vi "GEA2 Loop Check.vi"() -> ()   [LabVIEW 2016]
uses:
  LabVIEW GEA2 Toolkit v1.0.0.0/library/GEA2_Toolkit.lvlib
  HEWH/Type Definitions/GEA2 Commands.ctl
panel:
  out "min value":dbl
  out "max value":dbl
  out "Elapsed Time (sec)":dbl format="%.2f"
  in  "millisecond multiple":u32=1000
  out "T2(TankSensor)":dbl
  in  "stop":bool
  out "appended array":string[][](array[string])
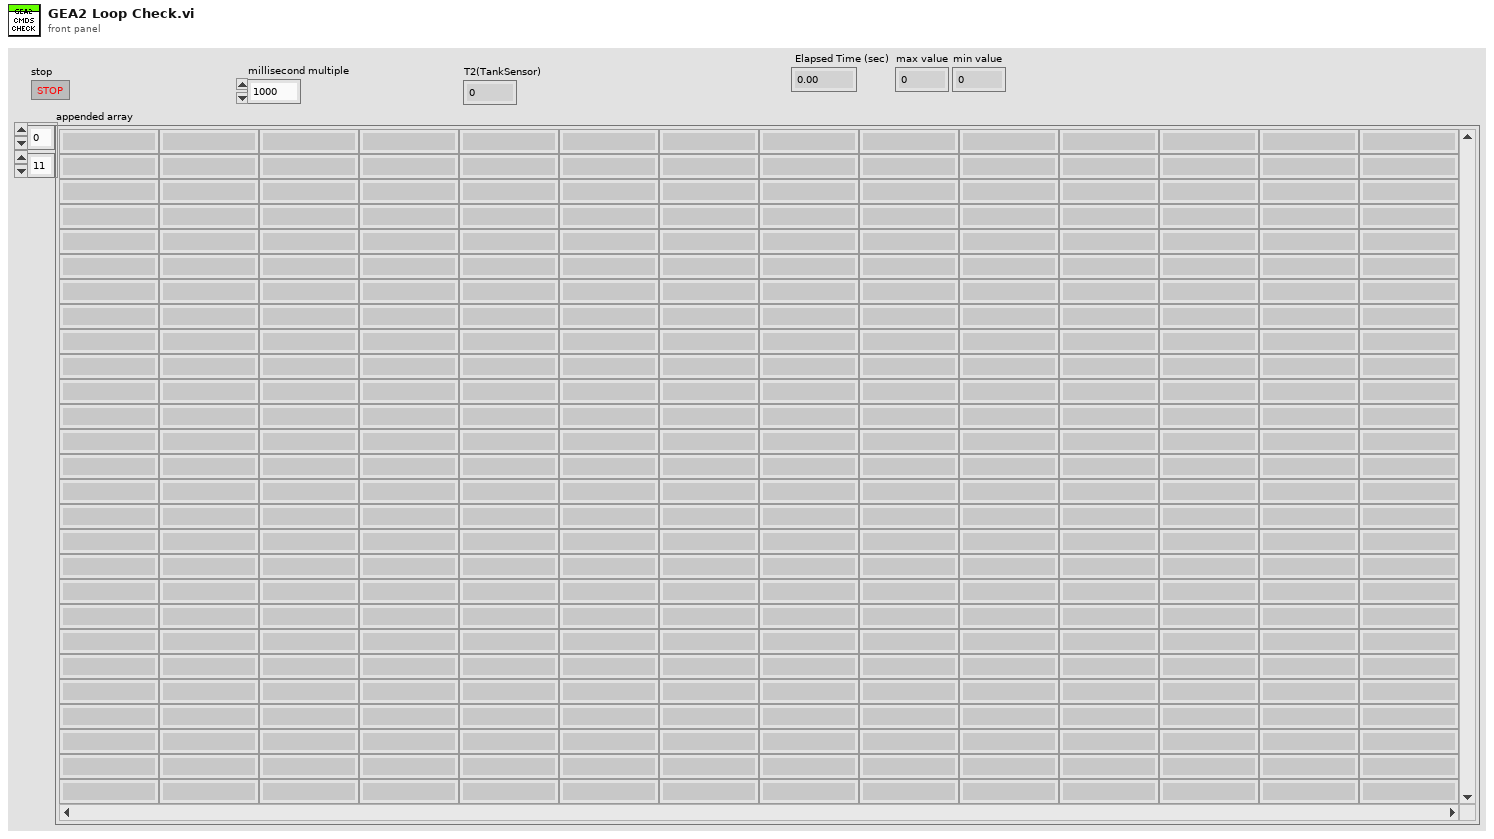
[diagram p1: front panel]
types:
  T1 = typedef "GEA2 Commands.ctl" = enum16{"CMD_CANCEL_EEV_POSITION", "CMD_CLEAR_ENERGY_USAGE_CTRS", "CMD_CLEAR_FAULT_COUNTS", "CMD_CLEAR_OVERRIDE_STATUS", "CMD_COMP_OFF", "CMD_COMP_ON", "CMD_DSM_OVERRIDES", "CMD_EEV_POSITION", "CMD_ENTER_EXIT_FCT_MODE", "CMD_ENTER_FACT_MODE", "CMD_HP_RUN_6MIN", "CMD_INITIATE_REMOTE_DSM_OVERRIDE", "CMD_LE_2_SECONDS", "CMD_REFRESH_SERVICE_TIMEOUTS", "CMD_RESET", "CMD_RESET_FILTER_TIMES", "CMD_RESTORE_EEPROM_DEFAULTS", "CMD_RQST_LED_STATUS", "CMD_SET_AMBIENT_THRESH_1", "CMD_SET_AMBIENT_THRESH_2", "CMD_SET_AMBIENT_THRESH_3", "CMD_SET_CURRENTS", "CMD_SET_EEV_DRIVE_LINES", "CMD_SET_EEV_STOP_POSITION", "CMD_SET_LEDS", "CMD_SET_MODEL_NUMBER", "CMD_SET_PID_I_DENOM_OVER_THR", "CMD_SET_PID_I_DENOM_UNDER_THR", "CMD_SET_PID_LOW_SH_TARGET", "CMD_SET_PID_MID_SH_TARGET", "CMD_SET_PID_P_DENOMINATOR", "CMD_SET_SERIAL_NUMBER", "CMD_SET_START_POS_OVER_THR", "CMD_SET_START_POS_UNDER_THR", "CMD_TOGGLE_FAN", "CMD_TOGGLE_LE_SERV", "CMD_TOGGLE_SERVICE_MODE", "CMD_TOGGLE_UE_SERV", "CMD_TURN_ON_OFF_DLB", "CMD_UE_2_SECONDS", "CMD_UPDATE_DSM_LEVEL", "CMD_UPDATE_MODE", "CMD_WRITE_SETPOINTS", "REQ_READ_KEY_STATUS", "REQ_SYSTEM_MODE", "RQST_CURRENT_PID_SH_TARGET", "RQST_DATA_FROM_DATA_FLASH", "RQST_DATA_FROM_MEMORY", "RQST_DSM_OVERRIDE_STATUS", "RQST_HEM_KWH_DATA", "RQST_HYPERTERM_OUTPUT_DATA", "RQST_IDLB_RESISTANCE", "RQST_MODEL_NUMBER", "RQST_MODEL_SELECT_AD_VALUE", "RQST_OTHER_FAULT_COUNTS", "RQST_OVERRIDE_STATUS", "RQST_PID_PARAMETERS", "RQST_READ_PERSONALITY", "RQST_SERIAL_NUMBER", "RQST_SERVICE_ERROR_CODES", "RQST_Software_Version", "RQST_SS_FAULT_COUNTS", "RQST_STATUS_QUERY", "RQST_STD_ELEC_RANGE", "RQST_SUPPORTED_MODES", "RQST_T2_RESISTANCE", "RQST_T3B_RESISTANCE", "RQST_T4_RESISTANCE", "RQST_T5_RESISTANCE", "RQST_TEMP_RANGE", "RQST_VACATION_RANGE", "RQST_WATER_CAPACITY"}
  T2 = typedef "GEA2_Toolkit.lvlib/Data In.ctl" = cluster{"Source":u8, "Destination":u8, "Command":u8, "Message":string}
  T3 = typedef "GEA2_Toolkit.lvlib/Data Out.ctl" = cluster{"Source":u8, "Destination":u8, "Command":u8, "Length":u8, "CRC":u16, "Message":string}
  T4 = typedef "ViperHawk Data.ctl" = cluster{"GEA Diagnostic Data - Washer":T5, "Software Version":T6, "Debug Search Parameters":T7, "Message Count":i32, "Number of Messages":i32, "Partial Message String":string, "Full Message to Save":string, "Board ID":string, "Board Index":i32, "Source Address":u8, "Destination Address":u8, "Data to send":u8[], "ReceivedData":u8[], "Debug/GEA Data":string[], "Command":u8, "GEA2 Reference Out":refnum<k24>, "GEA2 Event Registration":refnum<event-registration>, "Bus Data":string, "GEA Data":string[][], "Network Variable Location":i32, "Water Heater GEA2 Data":T8}
  T5 = typedef "ViperHawk Diagnostic Data.ctl" = cluster{"Speed (RPM)":u32, "Load Size":u32, "Temperature":u32, "Water Pressure":dbl, "Detergent":u32, "Fabric Softener":u32, "Tub Direction":string, "Detergent Valve":bool, "Fabric Softener Valve":bool, "Recirculating Pump":bool, "Drain Valve":bool, "Hot Valve":bool, "Cold Valve":bool, "Lid Closed Status":string, "Lid Lock Status":string, "Error Count":u32, "IGBT Temperature (Deg C)":u32, "Motor Speed":u32, "Latched OOB":u32, "Raw OOB":u32, "Plaster Status":u32, "Inverter Power (W)":u32, "Target Speed(BRPM)":u32, "Latched Agitate Motor Temp (Deg C)":u32, "Current Motor Temp (Deg C)":u32, "Profiler Status":string, "Current Inverter Action":string, "Error Codes":string, "Lid Locked":bool, "Lid Closed":bool, "9E Diagnostic Data":cluster{"Total Cycle Time (Min)":u32, "Total Cycle Count (Current)":u16, "Total Error Count":u16, "Machine Error History":u32, "Washer UI History":u32, "Inverter Error History":u32, "Cycle Storage Limit":u8, "Error Storage Limit":u8, "Cycle Pages Supported":u8, "Error Pages Supported":u8, "Inverter Reset Count":u16}, "9F Diagnostic Data":cluster{"Cycle Buffer Index":string, "Page Number":string, "Total Cycle Count":u32, "Delay Start Time":u32, "Stain Selected":string, "Selected Cycle":u32, "eWash":string, "Soil Level":string, "Temperature":string, "Overnight Ready":string, "Spin Setting":string, "Control Lock Status":string, "Stain Remover":string, "Steam Assist":string, "My Cycle":string, "PreWash":string, "Debug Log Enabled":string, "Rinse":string, "Signal Level":string, "PreSoak":string}}
  T6 = typedef "Save File.lvlib/Save File Software Version.ctl" = cluster{"Critical Major SW Version":string, "Critical Minor SW Version":string, "Major SW Version":string, "Minor SW Version":string, "Parametric Data Ver. Major":string, "Parametric Data Ver. Minor":string, "Diagnostics Data Ver. Major":string, "Diagnostics Data Ver. Minor":string, "Current Personality Setting":string}
  T7 = typedef "ViperHawk Search Control.ctl" = cluster{"Pause":string[], "Run":string[], "EOC":string[], "Error Codes":string[]}
  T8 = typedef "GEA2 Commands WaterHeater GEA2 Data.ctl" = cluster{"GEA2 Label Array":string[], "PID_PARAMETERS":string[][], "SUPPORTED_MODES":string[][], "Button Status":T9, "Status Query":T10, "Service Error Codes":T11, "HEM_KWH_DATA":string[][], "OTHER_FAULT_COUNTS":string[][], "GEA2 Raw Message":string, "Hyperterminal Data":cluster{"Source":u8, "Destination":u8, "Command":u8, "Length":u8, "CRC":u16, "UE - state (1/0 on off)":u8, "LE - state (1/0 on off)":u8, "Comp - state (1/0 on off)":u8, "Fan  - state (1/0 on off)":u8, "Setpoint Deg F":i32, "T2(TankSensor)":dbl, "T3A(EvapIn)":dbl, "T3B(EvapOut)":dbl, "T4(CompressorDischarge)":dbl, "T5(Ambient)":dbl, "Current":dbl, "Voltage (Volts)":u16, "EEV Position (0-480)":u16, "Reason for last heating cycle termination":u16, "Reason Data word 1":string, "Reason Data word 2":string, "Reason Data word 3":string, "Reason Data word 4":string, "SW Debug Data":string, "Flow Events (Bit Encoded)":u16, "Heating Control Mode":u16}, "Extra Data":cluster{"Water Capacity (Gallons)":u32, "Max Vacation Duration Days":u32, "Min Vacation Duration Days":u32, "Max Set Point (Deg F)":u32, "Min Set Point (Deg F)":u32, "T5 Resistance":u32, "T4 Resistance":u32, "T3B Resistance":u32, "T2 Resistance":u32, "STD_ELEC_RANGE":string, "SS_FAULT_COUNTS":string, "SERIAL_NUMBER":string, "READ_PERSONALITY":u8, "RQST_OVERRIDE_STATUS":string, "MODEL_SELECT_AD_VALUE":u32, "MODEL NUMBER":string, "IDLB_RESISTANCE":u32, "DSM Override Status":string, "RQST_DATA_FROM_Memory":string, "RQST_DATA_FROM_DATA_FLASH":string, "RQST_CURRENT_PID_SH_TARGET":u16, "Unit System Mode":string}}
  T9 = typedef "GEA2 Commands Button Status.ctl" = cluster{"Switch 1":bool, "Switch 2":bool, "Switch 3":bool, "Switch 4":bool, "Switch 5":bool, "Switch 6":bool, "Switch 7":bool, "Switch 8":bool, "Switch 9":bool, "Switch 10":bool, "Switch 11":bool, "Switch 12":bool, "Switch 13":bool, "Switch 14":bool, "Switch 15":bool, "Switch 16":bool}
  T10 = typedef "GEA2 Commands Status Query.ctl" = cluster{"Days Remaining (For Std Electric and Vacation)":u8, "Unit Status":string, "Current Tank Temp in Deg F":u8, "Current Setpoint in Deg F":u8, "Filter Status (% used)":u8, "Fallback Status (Fallback heating mode)":string, "Fallback Temp":u8, "\"Set Mode\" Selection":string}
  T11 = typedef "GEA2 Commands Service Error Codes.ctl" = cluster{"Reserved":bool, "Reserved 1":bool, "Reserved 2":bool, "Reserved 3":bool, "Reserved 4":bool, "Reserved 5":bool, "Reserved 6":bool, "Reserved 7":bool, "DataFlash Fail Status":bool, "Stuck Key Fail Status":bool, "Dry Tank Fail Status":bool, "Miswire Fail Status":bool, "Reserved 8":bool, "Reserved 9":bool, "Reserved 10":bool, "Reserved 11":bool, "UE Fail Status":bool, "LE Fail Status":bool, "Filter Fail Status":bool, "T3A Fail Status":bool, "T3B Fail Status":bool, "T4 Fail Status":bool, "T5 Fail Status":bool, "T2 Fail Status":bool, "SS Cond A Status":bool, "SS Cond B Status":bool, "SS Cond C Status":bool, "SS Cond D Status":bool, "SS Cond E Status":bool, "SS Cond F Status":bool, "SS Fan Status":bool, "CMP Fail Status":bool}
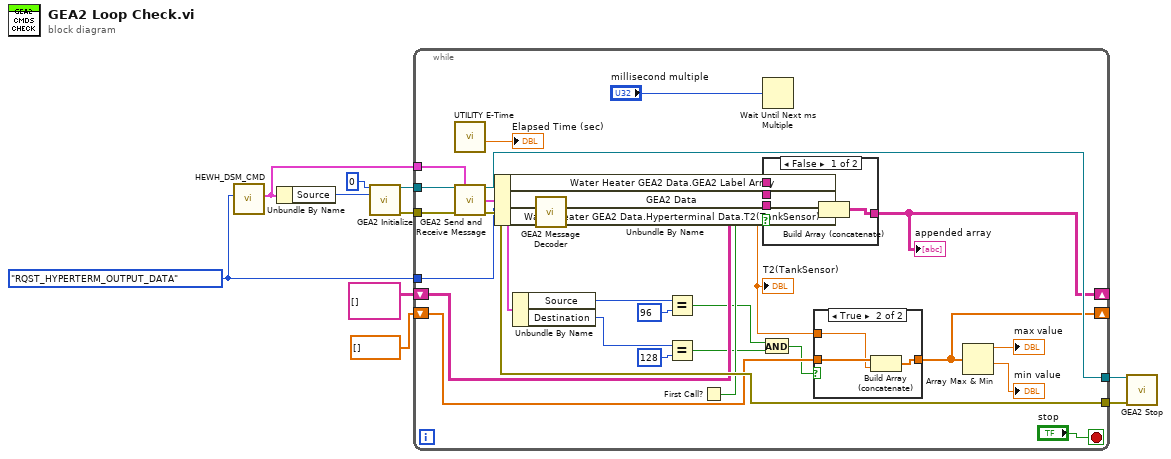
[diagram p0: block diagram]
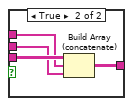
[diagram p3: hidden frame]
diagram:
  w4 = GEA2_Commands."RQST_HYPERTERM_OUTPUT_DATA" ("GEA2 Commands and Requests")
  n1 = call "HEWH_DSM_CMD.vi"("GEA2 Commands and Requests"=w4) -> ("Input Data"=w2:T2)  [unwired: 8 in, 1 out]
  n2 = Unbundle By Name(w2) -> ("Source"=w10:u8)
  n3 = call "GEA2 Initialize.vi"("Board Index"=0, "Source Address"=w10) -> ("GEA2 Reference Out"=w8:refnum<k24>, "error out"=w6:errorcluster)  [unwired: 11 in, 1 out]
  n4 = while {
    tunnel: w8 -> [w38]
    tunnel: [w37] -> w7
    tunnel: w6 -> [w36]
    tunnel: [w35] -> w5
    tunnel: w4 -> [w34]
    shift-right: [w31] -> _
    shift-left: string[][] [] -> [w33]
    tunnel: w2 -> [w29]
    shift-right: [w22] -> _
    shift-left: dbl[] [] -> [w24]
    stop <- "stop" stop-if-true
    n5 = call "UTILITY E-Time.vi"() -> ("Elapsed Time (sec)"=→"Elapsed Time (sec)":dbl)  [unwired: 9 in, 2 out]
    n6 = call "GEA2 Send and Receive Message.vi"("GEA2 Reference In"=w38, "Input Data"=w29, "Error In"=w36) -> ("GEA2 Reference Out"=w37:refnum<k24>, "Converted Data Out"=w18:T3, "Error Out"=w35:errorcluster)  [unwired: 7 in, 3 out]
    n7 = Unbundle By Name(w18) -> ("Source"=w17:u8, "Destination"=w15:u8)
    n8 = call "GEA2 Message Decoder.vi"("GEA2 Commands and Requests"=w34, "Coverted Data Out"=w18) -> ("GEA Information Out"=w32:T4)  [unwired: 9 in]
    n9 = Unbundle By Name(w32) -> ("Water Heater GEA2 Data.GEA2 Label Array"=w27:string[], "GEA2 Data"=w19:string[], "Water Heater GEA2 Data.Hyperterminal Data.T2(TankSensor)"=w23:dbl)
    "T2(TankSensor)" <- w23
    n10 = Equal?(x=w17, y=u8 96) -> (x = y?=w13:bool)
    n11 = Equal?(x=w15, y=u8 128) -> (x = y?=w12:bool)
    n12 = First Call?() -> (First Call?: T/F=w26:bool)
    n13 = And(x=w13, y=w12) -> (x .and. y?=w11:bool)
    n14 = Wait Until Next ms Multiple(millisecond multiple="millisecond multiple") -> ()  [unwired: 1 out]
    n15 = case shown="False" w26 {
      tunnel: w33 -> [w45 w49]
      tunnel: [w44 w48] -> w31
      tunnel: w19 -> [w43 w47]
      tunnel: w27 -> [_ w46]
      frame False {
        n16 = Build Array (concatenate)(w45, w43) -> (w44:string[][])
      }
      frame True {
        n17 = Build Array (concatenate)(w49, w46, w47) -> (w48:string[][])
      }
    }
    "appended array" <- w31
    n18 = case shown="True" w11 {
      tunnel: w24 -> [w39 w42]
      tunnel: w23 -> [_ w41]
      tunnel: [w39 w40] -> w22
      frame False {
      }
      frame True {
        n19 = Build Array (concatenate)(w42, w41) -> (w40:dbl[])
      }
    }
    n20 = Array Max & Min(array=w22) -> (max value=→"max value":dbl, min value=→"min value":dbl)  [unwired: 2 out]
  }
  n21 = call "GEA2 Stop.vi"("GEA2 Reference Out"=w7, "Error In"=w5) -> ()  [unwired: 13 in, 1 out]
